vi "PDW 2 graph.vi"(8 "error in (no error)":errorcluster, 9 "color plate":T3, 10 "PDW":cluster{"PDW":T1[], "Ton":dbl[]} {"PDW"."frequency shift" format="%#_12f"}, 11 "device_type in":refnum<class "device_type.lvclass">) -> (0 "error out":errorcluster, 1 "color":u32[](array[numeric]), 2 "graph":cluster{dbl[], dbl[]}[](array[cluster]), 3 "device_type out":refnum<class "device_type.lvclass">)   [LabVIEW 2021, in "device_type.lvclass"]
uses:
  device_type.lvclass
  pulse_tx_vis/pdw.ctl
  pulse_tx_vis/CTL/mode_type.ctl
  device_type.lvclass/device_type.ctl
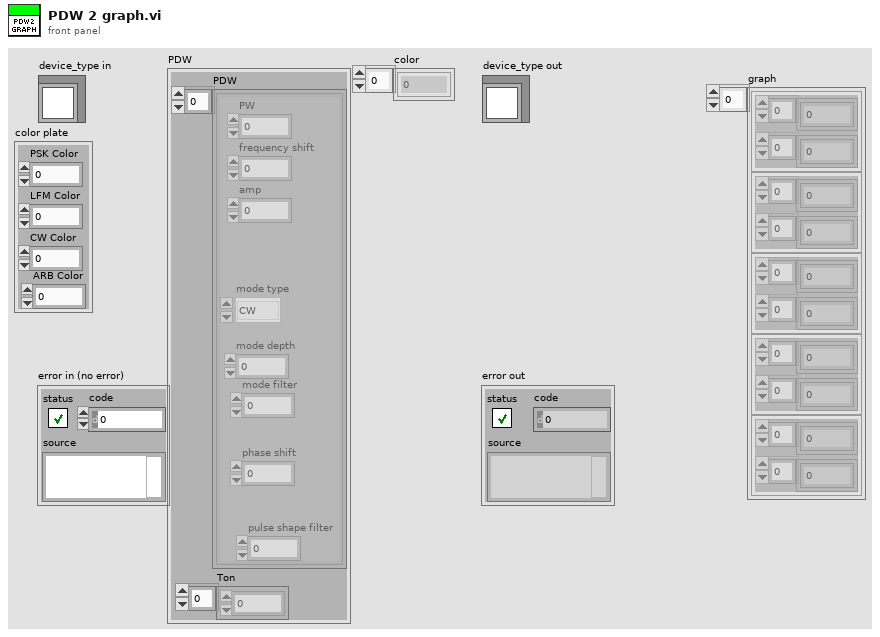
[diagram p1: front panel]
types:
  T1 = typedef "pdw.ctl" = cluster{"PW":u32, "frequency shift":fxp<+/-,48,0>, "amp":fxp<+/-,18,1>, "mode type":T2, "mode depth":u32, "mode filter":u8, "phase shift":fxp<+/-,16,1>, "pulse shape filter":u8}
  T2 = typedef "mode_type.ctl" = enum8{"CW", "from memory 1", "NC - cw", "LFM", "BPSK", "QPSK"}
  T3 = cluster{"PSK Color":u32, "LFM Color":u32, "CW Color":u32, "ARB Color":u32}
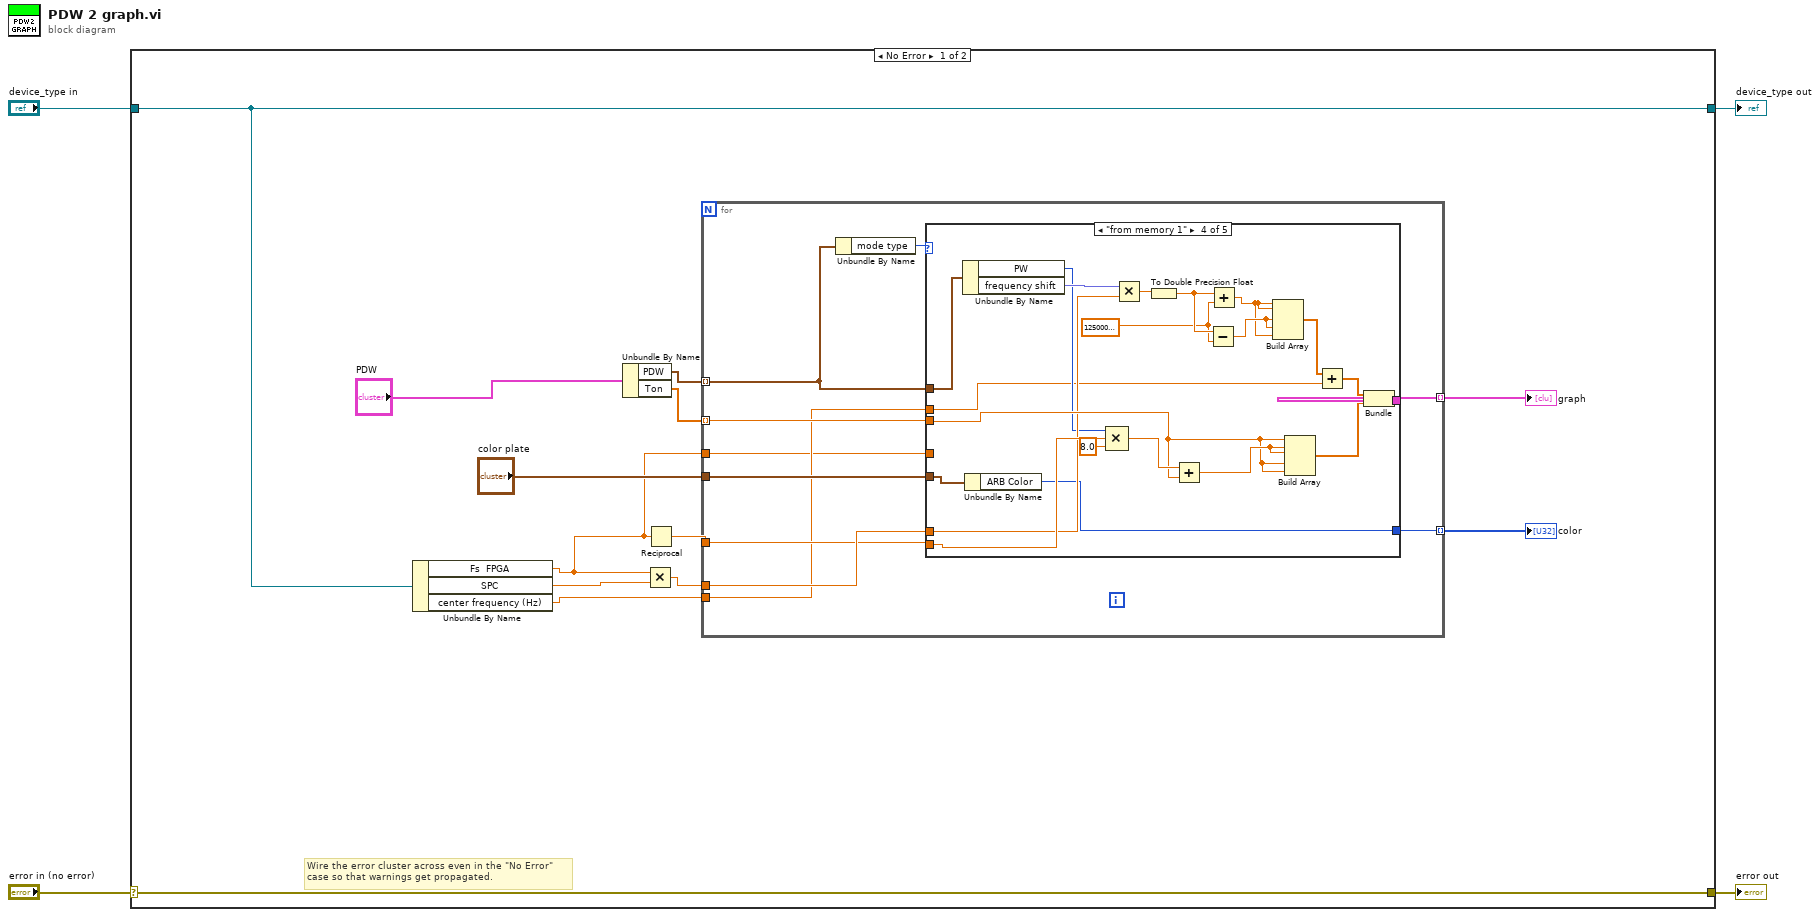
[diagram p0: block diagram]
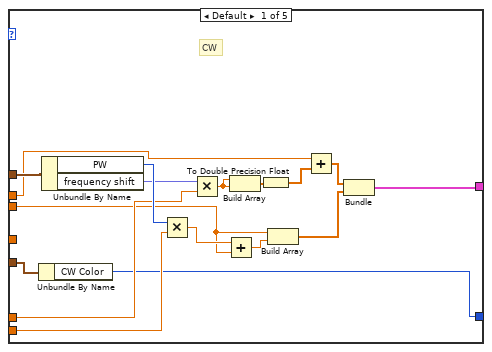
[diagram p2: hidden frame]
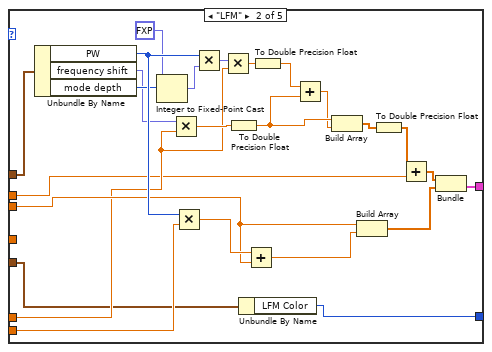
[diagram p3: hidden frame]
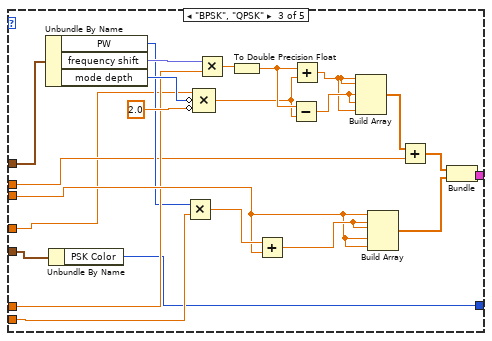
[diagram p4: hidden frame]
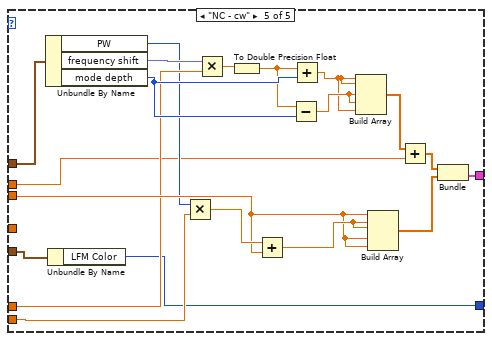
[diagram p5: hidden frame]
diagram:
  n1 = case shown="No Error" "error in (no error)" {
    selector: "error in (no error)" -> [w17 w135]
    tunnel: [w17 w135] -> w3
    tunnel: [w5 w134] -> w1
    tunnel: "device_type in" -> [w5 w134]
    frame No Error {
      # "Wire the error cluster across even in the \"No Error\"\ncase so that warnings get propagated."
      n2 = Unbundle By Name(w5) -> ("Fs  FPGA"=w6:dbl, "SPC"=w8:dbl, "center frequency (Hz)"=w7:dbl)
      n3 = Unbundle By Name("PDW") -> ("PDW"=w14:T1[], "Ton"=w15:dbl[])
      n4 = Multiply(x=w6, y=w8) -> (x*y=w12:dbl)
      n5 = Reciprocal(x=w6) -> (1/x=w9:dbl)
      n6 = for {
        tunnel: w12 -> [w26]
        tunnel: w9 -> [w25]
        tunnel: [w24] -> w10 mode=indexing
        tunnel: [w23] -> w11 mode=indexing
        tunnel: w14 -> [w22] mode=indexing
        tunnel: w15 -> [w21] mode=indexing
        tunnel: "color plate" -> [w20]
        tunnel: w7 -> [w19]
        tunnel: w6 -> [w18]
        n7 = Unbundle By Name(w22) -> ("mode type"=w27:T2)
        n8 = case shown="\"from memory 1\"" w27 {
          tunnel: w21 -> [w34 w62 w87 w108 w128]
          tunnel: w22 -> [w44 w65 w89 w110 w130]
          tunnel: w26 -> [w41 w54 w84 w107 w126]
          tunnel: w25 -> [w40 w66 w90 w111 w131]
          tunnel: [w38 w67 w76 w100 w119] -> w24
          tunnel: [w29 w46 w72 w96 w114] -> w23
          tunnel: w20 -> [w30 w47 w73 w97 w116]
          tunnel: w19 -> [w28 w45 w71 w95 w115]
          tunnel: w18 -> [_ _ w70 _ _]
          frame Default {
            # "CW"
            n9 = Unbundle By Name(w30) -> ("CW Color"=w29:u32)
            n10 = Unbundle By Name(w44) -> ("PW"=w43:u32, "frequency shift"=w42:fxp<+/-,48,0>)
            n11 = Multiply(x=w43, y=w40) -> (x*y=w35:dbl)
            n12 = Multiply(x=w42, y=w41) -> (x*y=w39:dbl)
            n13 = Add(x=w35, y=w34) -> (x+y=w33:dbl)
            n14 = Build Array(w39, w39) -> (w36:dbl[])
            n15 = To Double Precision Float(number=w36) -> (double precision float=w32:dbl[])
            n16 = Build Array(w34, w33) -> (w37:dbl[])
            n17 = Add(x=w28, y=w32) -> (x+y=w31:dbl[])
            n18 = Bundle(w31, w37) -> (w38:cluster{dbl[], dbl[]})  [unwired: 1 in]
          }
          frame "LFM" {
            n19 = Unbundle By Name(w65) -> ("PW"=w64:u32, "frequency shift"=w56:fxp<+/-,48,0>, "mode depth"=w59:u32)
            n20 = Integer to Fixed-Point Cast(fixed-point type=fxp<+,32,-16> 0.0, integer=w59) -> (fixed-point=w55:fxp<+,32,-16>)
            n21 = Multiply(x=w56, y=w54) -> (x*y=w57:dbl)
            n22 = Multiply(x=w64, y=w66) -> (x*y=w63:dbl)
            n23 = Multiply(x=w64, y=w55) -> (x*y=w53:fxp<+,64,16>)
            n24 = Multiply(x=w53, y=w54) -> (x*y=w58:dbl)
            n25 = To Double Precision Float(number=w57) -> (double precision float=w52:dbl)
            n26 = Unbundle By Name(w47) -> ("LFM Color"=w46:u32)
            n27 = Add(x=w63, y=w62) -> (x+y=w61:dbl)
            n28 = To Double Precision Float(number=w58) -> (double precision float=w51:dbl)
            n29 = Add(x=w51, y=w52) -> (x+y=w50:dbl)
            n30 = Build Array(w52, w50) -> (w68:dbl[])
            n31 = Build Array(w62, w61) -> (w69:dbl[])
            n32 = To Double Precision Float(number=w68) -> (double precision float=w49:dbl[])
            n33 = Add(x=w49, y=w45) -> (x+y=w48:dbl[])
            n34 = Bundle(w48, w69) -> (w67:cluster{dbl[], dbl[]})  [unwired: 1 in]
          }
          frame "BPSK", "QPSK" {
            n35 = Unbundle By Name(w89) -> ("PW"=w81:u32, "frequency shift"=w83:fxp<+/-,48,0>, "mode depth"=w86:u32)
            n36 = Unbundle By Name(w73) -> ("PSK Color"=w72:u32)
            n37 = Multiply(x=w81, y=w90) -> (x*y=w91:dbl)
            n38 = Compound Arithmetic op=MULTIPLY(w70, invert w86, invert 2.0 ("value")) -> (w79:dbl)
            n39 = Multiply(x=w83, y=w84) -> (x*y=w82:dbl)
            n40 = To Double Precision Float(number=w82) -> (double precision float=w80:dbl)
            n41 = Add(x=w91, y=w87) -> (x+y=w88:dbl)
            n42 = Subtract(x=w80, y=w79) -> (x-y=w78:dbl)
            n43 = Add(x=w80, y=w79) -> (x+y=w77:dbl)
            n44 = Build Array(w77, w77, w78, w78, w77) -> (w75:dbl[])
            n45 = Build Array(w87, w88, w88, w87, w87) -> (w92:dbl[])
            n46 = Add(x=w75, y=w71) -> (x+y=w74:dbl[])
            n47 = Bundle(w74, w92) -> (w76:cluster{dbl[], dbl[]})  [unwired: 1 in]
          }
          frame "from memory 1" {
            w93 = 12500000.0 ("y")
            n48 = Unbundle By Name(w110) -> ("PW"=w104:u32, "frequency shift"=w106:fxp<+/-,48,0>)
            n49 = Unbundle By Name(w97) -> ("ARB Color"=w96:u32)
            n50 = Compound Arithmetic op=MULTIPLY(w104, w111, 8.0 ("value")) -> (w112:dbl)
            n51 = Multiply(x=w106, y=w107) -> (x*y=w105:dbl)
            n52 = To Double Precision Float(number=w105) -> (double precision float=w103:dbl)
            n53 = Add(x=w112, y=w108) -> (x+y=w109:dbl)
            n54 = Subtract(x=w103, y=w93) -> (x-y=w102:dbl)
            n55 = Add(x=w103, y=w93) -> (x+y=w101:dbl)
            n56 = Build Array(w101, w101, w102, w102, w101) -> (w99:dbl[])
            n57 = Build Array(w108, w109, w109, w108, w108) -> (w113:dbl[])
            n58 = Add(x=w99, y=w95) -> (x+y=w98:dbl[])
            n59 = Bundle(w98, w113) -> (w100:cluster{dbl[], dbl[]})  [unwired: 1 in]
          }
          frame "NC - cw" {
            n60 = Unbundle By Name(w130) -> ("PW"=w123:u32, "frequency shift"=w125:fxp<+/-,48,0>, "mode depth"=w127:u32)
            n61 = Unbundle By Name(w116) -> ("LFM Color"=w114:u32)
            n62 = Multiply(x=w123, y=w131) -> (x*y=w132:dbl)
            n63 = Multiply(x=w125, y=w126) -> (x*y=w124:dbl)
            n64 = To Double Precision Float(number=w124) -> (double precision float=w122:dbl)
            n65 = Add(x=w132, y=w128) -> (x+y=w129:dbl)
            n66 = Subtract(x=w122, y=w127) -> (x-y=w121:dbl)
            n67 = Add(x=w122, y=w127) -> (x+y=w120:dbl)
            n68 = Build Array(w120, w120, w121, w121, w120) -> (w118:dbl[])
            n69 = Build Array(w128, w129, w129, w128, w128) -> (w133:dbl[])
            n70 = Add(x=w118, y=w115) -> (x+y=w117:dbl[])
            n71 = Bundle(w117, w133) -> (w119:cluster{dbl[], dbl[]})  [unwired: 1 in]
          }
        }
      }
      "color" <- w11
      "graph" <- w10
    }
    frame Error {
    }
  }
  "error out" <- w3
  "device_type out" <- w1
